vi "Inspection.vi"(8 "Error In":errorcluster, 11 "Data In":T2={"Console log"="", "GUI_Events"={"To_GUI-Producer"=refnum, "To_GUI-Error_message"=refnum, "To_GUI-msg_list"=refnum, "To_GUI-Session"=refnum, "To_GUI-Pre-Session"=refnum, "To_GUI-Consumer"=refnum}, "Function_Queue"={"Queue_MIDI_Handler"=refnum, "Queue_Session"=refnum, "Queue_Producer"=refnum, "Queue_Consumer"=refnum}, "Timout-Time[ms]"=0, "MIDI-Messages"=[], "Com Session State"=enum."Active Session", "Result Data"={"Diff"=[], "Tx Byte"=[], "Rx Byte"=[], "Send Log"=[], "Parsed Data"={"Tx MIDI Tag"=[], "Tx MIDI Parsed Data"=[], "Tx Error"=[], "Tx Running States"=[], "Rx MIDI Tag"=[], "Rx MIDI Parsed Data"=[], "Rx Error"=[], "Rx Running States"=[], "Diff"=[]}}, "Get #"=[], "CPU(ms)"=0}) -> (0 "Error Out":errorcluster, 3 "Consumer Data":T11={"Queue_Consumer"=refnum, "Selected Consumer"=enum."Random", "Session Data"={"Tx-Data"=[], "Rx-Data"=[], "MIDI-Message log"=[{"Message Name"="", "Meta value"=0, "Datastring"="", "Datatype"=enum."No Data"}]}, "Timout-Time[ms]"=0, "To_GUI-Consumer"=refnum, "CPU(ms)"=0, "Console log"="", "MIDI Parse Data"={"MIDI-Bytes In"=[145, 60, 100], "MIDI Tag"=[], "MIDI Parsed Data"=[], "Iteration"=0, "Error?"=[], "Running States"=[], "Running Statusbyte"=0, "Running StatusString"="", "Third Byte Flag"=FALSE, "Current Byte"=0, "Sysex"="", "Expect Databyte"=FALSE}, "Session Inspection Data"={"Diff"=[], "Tx Byte"=[], "Rx Byte"=[], "Send Log"=[], "Parsed Data"={"Tx MIDI Tag"=[], "Tx MIDI Parsed Data"=[], "Tx Error"=[], "Tx Running States"=[], "Rx MIDI Tag"=[], "Rx MIDI Parsed Data"=[], "Rx Error"=[], "Rx Running States"=[], "Diff"=[]}}} {"MIDI Parse Data"."Current Byte" format="%.0x"; "MIDI Parse Data"."Running Statusbyte" format="%.0x"; "MIDI Parse Data"."MIDI-Bytes In" format="%.0x"})   [LabVIEW 2019]
doc: "Description of VI"
uses:
  Common/Controls/Application_Data.ctl
  Common/Controls/App_Events.ctl
  Common/Controls/App_Queues.ctl
  Common/Controls/Application_Message.ctl
  Common/Controls/Application_State.ctl
  MIDI/Controls/MIDI-Message_Array.ctl
  MIDI/Controls/MIDI-Message_Cluster.ctl
  MIDI/Controls/Meta_Commands.ctl
  Producer/Controls/Session_State.ctl
  Controls/Consumer_Result.ctl
  Controls/Parsed_Data.ctl
  Controls/Consumer_Data.ctl
  Controls/Consumer_States.ctl
  Controls/Transfer_Data.ctl
  Controls/Parser-data.ctl
  <vilib>/Utility/error.llb/DialogType.ctl
panel:
  out "Control Tab":T1(tab)
  out "Console Out":string
  out "Error Message":string
  out "VI-filename":string
  out "VI Path":path
  out "Code Size":u32
  out "Revision Number":u32
  in  "Tool Bar:Visible":bool
  in  "Tabs Visible?":bool
  out "VI-Name":string
  # "Add log!"
  # "Settings"
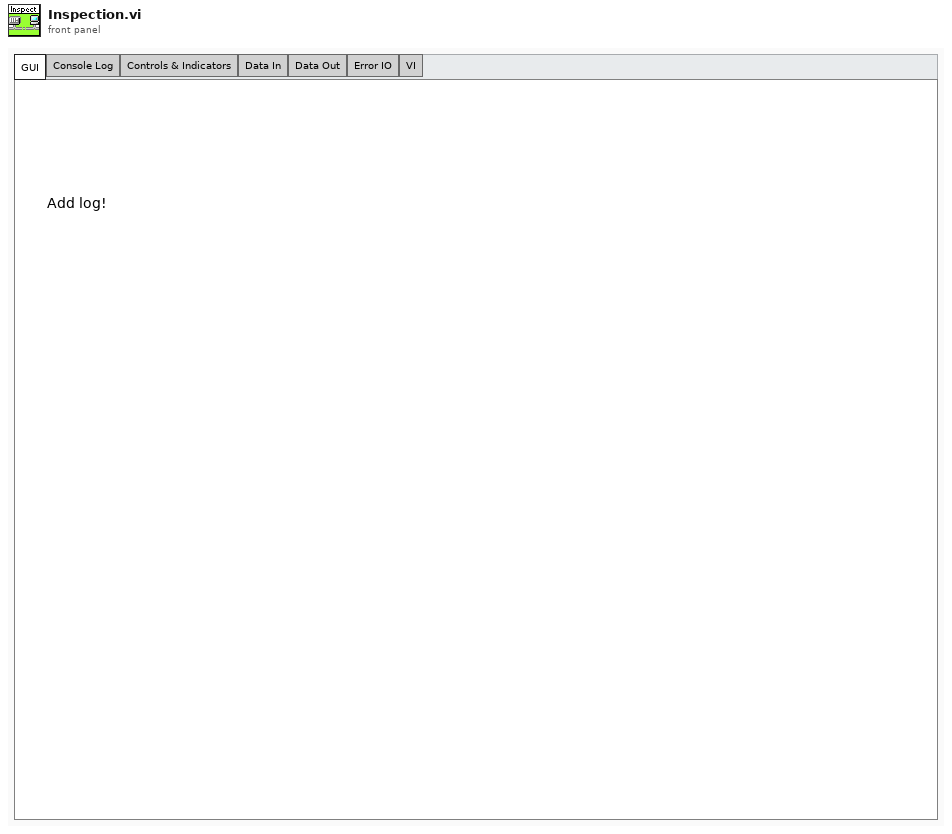
[diagram p1: front panel]
types:
  T1 = enum32{"GUI", "Console Log", "Controls & Indicators", "Data In", "Data Out", "Error IO", "VI"}
  T2 = typedef "Application_Data.ctl" = cluster{"Console log":string, "GUI_Events":T3, "Function_Queue":T4, "Timout-Time[ms]":i32, "MIDI-Messages":T5, "Com Session State":T8, "Result Data":T9, "Get #":bool[], "CPU(ms)":u32}
  T3 = typedef "App_Events.ctl" = cluster{"To_GUI-Producer":refnum<user-event>, "To_GUI-Error_message":refnum<user-event>, "To_GUI-msg_list":refnum<user-event>, "To_GUI-Session":refnum<user-event>, "To_GUI-Pre-Session":refnum<user-event>, "To_GUI-Consumer":refnum<user-event>}
  T4 = typedef "App_Queues.ctl" = cluster{"Queue_MIDI_Handler":refnum<queue>, "Queue_Session":refnum<queue>, "Queue_Producer":refnum<queue>, "Queue_Consumer":refnum<queue>}
  T5 = typedef "MIDI-Message_Array.ctl" = T6[]
  T6 = typedef "MIDI-Message_Cluster.ctl" = cluster{"Message Name":string, "Meta value":i32, "Datastring":string, "Datatype":T7}
  T7 = typedef "Meta_Commands.ctl" = enum16{"No Data", "Pause", "Loop", "Wait for Rx", "Delay", "Break", "MIDI"}
  T8 = typedef "Session_State.ctl" = enum16{"Wait to begin", "Active Session", "Pause", "Wait for Response", "Stop", "Restart", "Inspect", "Exit"}
  T9 = typedef "Consumer_Result.ctl" = cluster{"Diff":bool[], "Tx Byte":string[], "Rx Byte":string[], "Send Log":string[], "Parsed Data":T10}
  T10 = typedef "Parsed_Data.ctl" = cluster{"Tx MIDI Tag":string[], "Tx MIDI Parsed Data":string[], "Tx Error":bool[], "Tx Running States":string[], "Rx MIDI Tag":string[], "Rx MIDI Parsed Data":string[], "Rx Error":bool[], "Rx Running States":string[], "Diff":bool[]}
  T11 = typedef "Consumer_Data.ctl" = cluster{"Queue_Consumer":refnum<queue>, "Selected Consumer":T12, "Session Data":T13, "Timout-Time[ms]":i32, "To_GUI-Consumer":refnum<user-event>, "CPU(ms)":u32, "Console log":string, "MIDI Parse Data":T14, "Session Inspection Data":T9}
  T12 = typedef "Consumer_States.ctl" = enum16{"Random", "ECG", "Strech-Patch"}
  T13 = typedef "Transfer_Data.ctl" = cluster{"Tx-Data":i8[], "Rx-Data":i8[], "MIDI-Message log":T5}
  T14 = typedef "Parser-data.ctl" = cluster{"MIDI-Bytes In":u8[], "MIDI Tag":string[], "MIDI Parsed Data":string[], "Iteration":i32, "Error?":bool[], "Running States":string[], "Running Statusbyte":u8, "Running StatusString":string, "Third Byte Flag":bool, "Current Byte":u8, "Sysex":string, "Expect Databyte":bool}
  T15 = typedef "DialogType.ctl" = u16
  T16 = enum16{"open", "replace", "create", "open or create", "replace or create", "replace or create with confirmation"}
  T17 = typedef "Application_State.ctl" = enum16{"Idle", "Initiate", "MH Load Messages", "Prepare for Tx", "Settings", "Com Session", "Receive", "Data", "Uninitialize", "Quit Message", "Export Send"}
  T18 = typedef "Application_Message.ctl" = cluster{"Application State":T17, "Payload":variant}
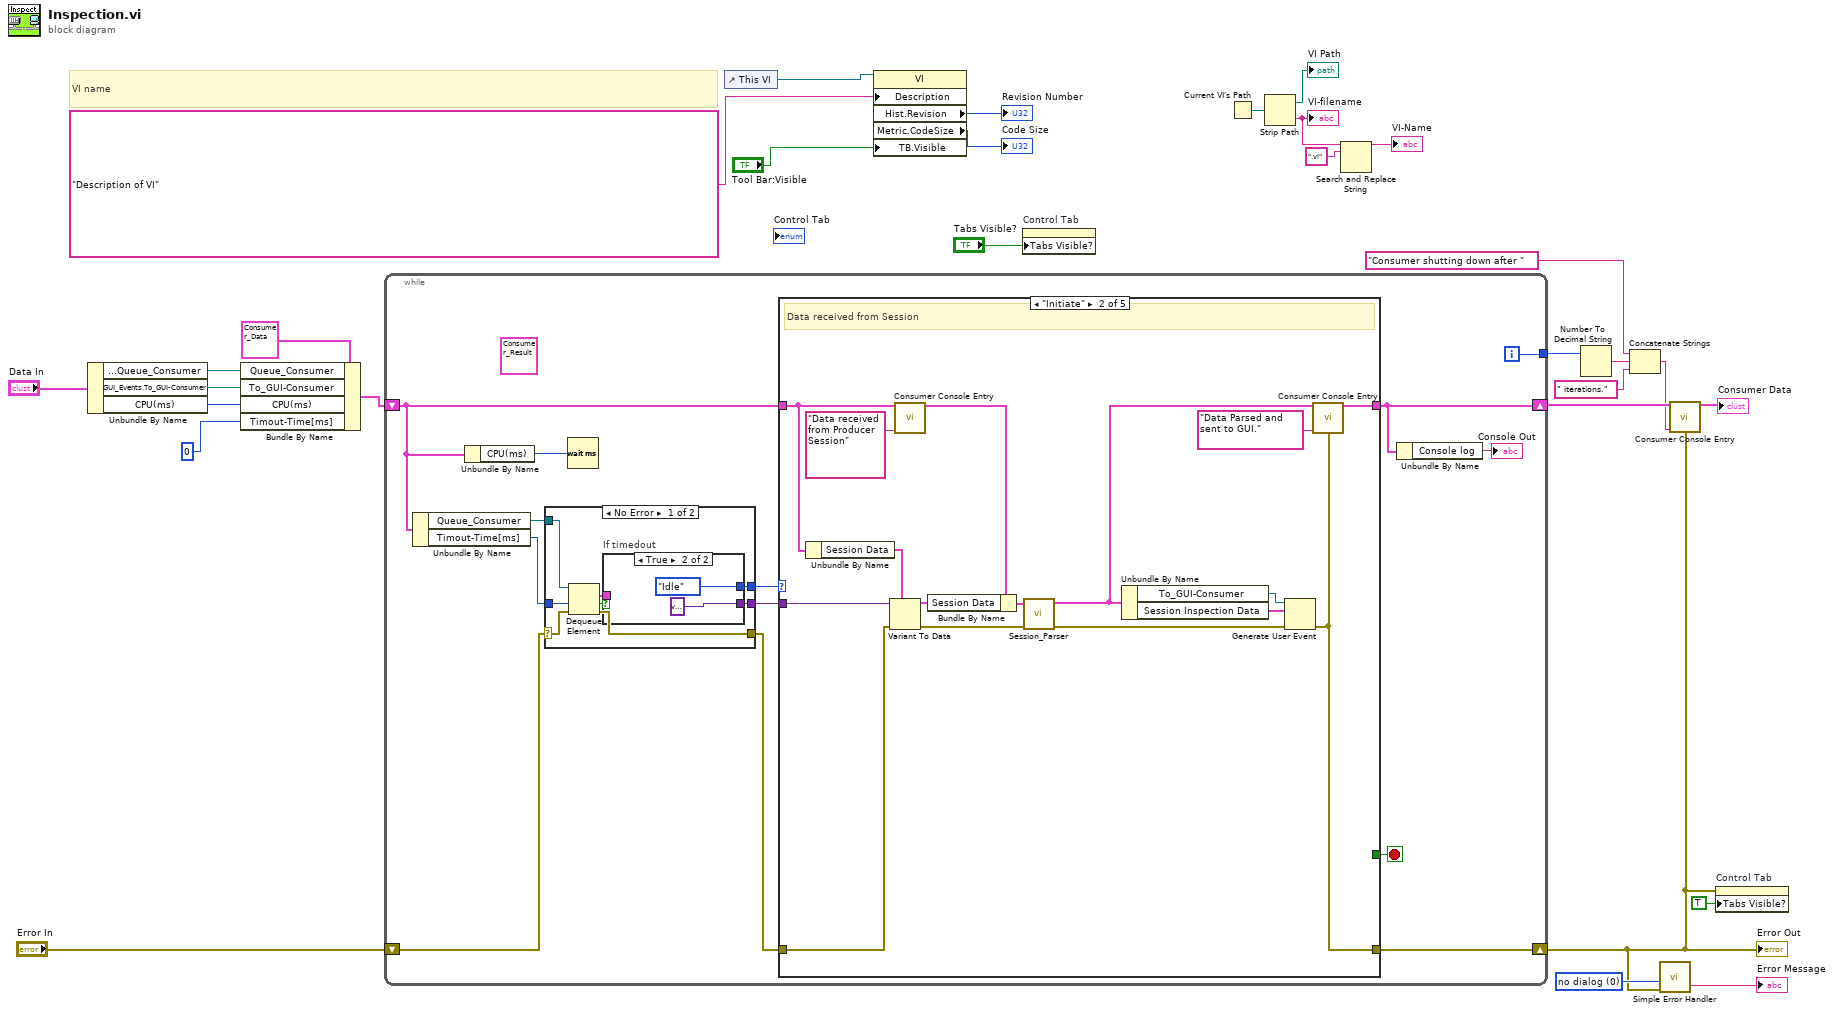
[diagram p0: block diagram]
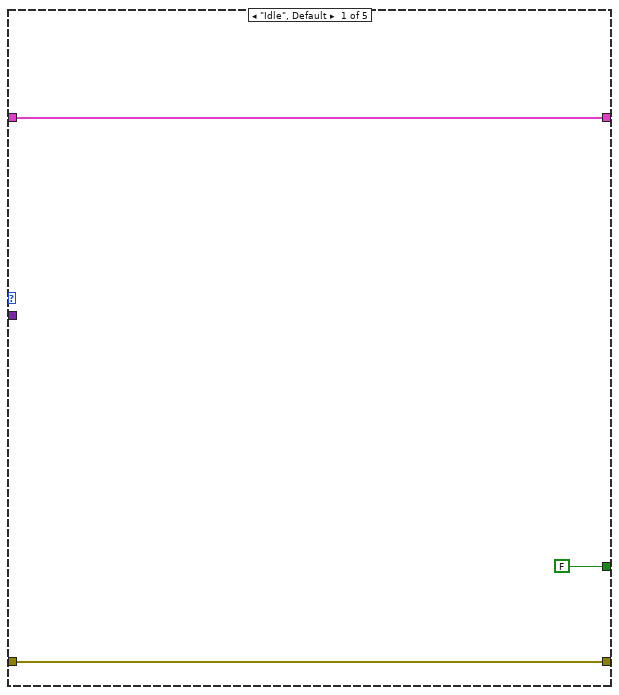
[diagram p2: hidden frame]
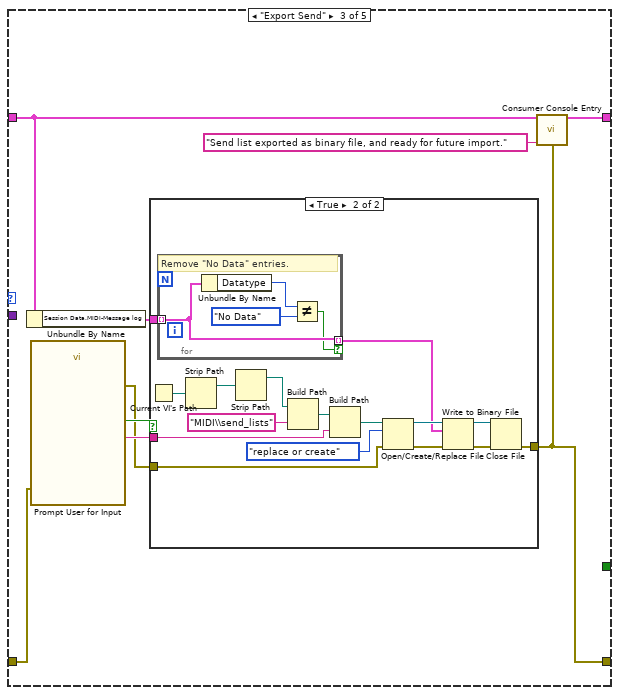
[diagram p3: hidden frame]
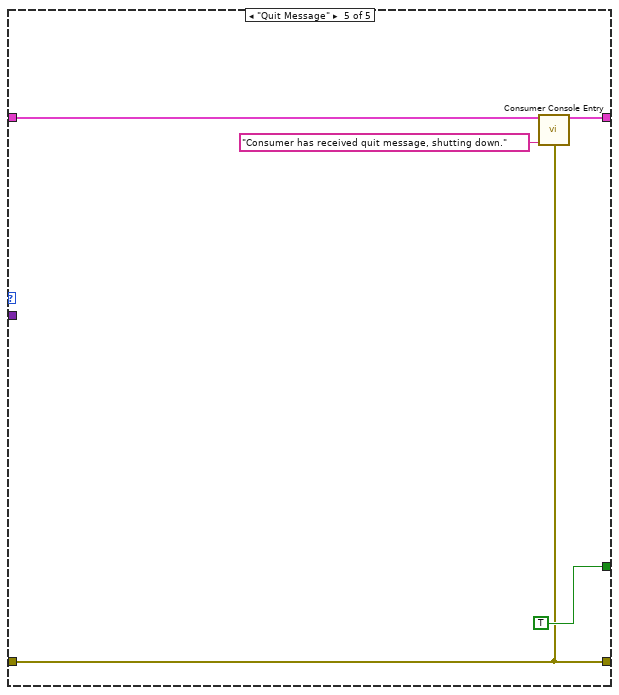
[diagram p6: hidden frame]
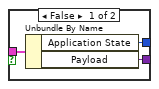
[diagram p7: hidden frame]
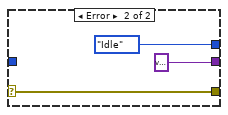
[diagram p8: hidden frame]
diagram:
  w21 = T15 0 items=["no dialog", "OK message", "continue or stop message", "OK message + warnings", "continue/stop + warnings"] ("type of dialog (OK msg:1)")
  # "VI name"
  n1 = Unbundle By Name("Data In") -> ("Function_Queue.Queue_Consumer"=w14:refnum<queue>, "GUI_Events.To_GUI-Consumer"=w11:refnum<user-event>, "CPU(ms)"=w9:u32)
  n2 = Bundle By Name(cluster=T11 {"Queue_Consumer"=refnum, "Selected Consumer"=enum."Random", "Session Data"={"Tx-Data"=[], "Rx-Data"=[], "MIDI-Message log"=[{"Message Name"="", "Meta value"=0, "Datastring"="", "Datatype"=enum."No Data"}]}, "Timout-Time[ms]"=0, "To_GUI-Consumer"=refnum, "CPU(ms)"=0, "Console log"="", "MIDI Parse Data"={"MIDI-Bytes In"=[145, 60, 100], "MIDI Tag"=[], "MIDI Parsed Data"=[], "Iteration"=0, "Error?"=[], "Running States"=[], "Running Statusbyte"=0, "Running StatusString"="", "Third Byte Flag"=FALSE, "Current Byte"=0, "Sysex"="", "Expect Databyte"=FALSE}, "Session Inspection Data"={"Diff"=[], "Tx Byte"=[], "Rx Byte"=[], "Send Log"=[], "Parsed Data"={"Tx MIDI Tag"=[], "Tx MIDI Parsed Data"=[], "Tx Error"=[], "Tx Running States"=[], "Rx MIDI Tag"=[], "Rx MIDI Parsed Data"=[], "Rx Error"=[], "Rx Running States"=[], "Diff"=[]}}} ("Consumer Data"), "Queue_Consumer"=w14, "To_GUI-Consumer"=w11, "CPU(ms)"=w9, "Timout-Time[ms]"=0) -> (w13:T11)
  n3 = while {
    shift-right: [w33] -> w7
    shift-left: w13 -> [w35]
    shift-right: [w38] -> w1
    shift-left: "Error In" -> [w40]
    tunnel: [w31] -> w4
    i -> [w31]
    stop <- w36 stop-if-true
    (unwired) T9 {"Diff"=[], "Tx Byte"=[], "Rx Byte"=[], "Send Log"=[], "Parsed Data"={"Tx MIDI Tag"=[], "Tx MIDI Parsed Data"=[], "Tx Error"=[], "Tx Running States"=[], "Rx MIDI Tag"=[], "Rx MIDI Parsed Data"=[], "Rx Error"=[], "Rx Running States"=[], "Diff"=[]}}
    n4 = Unbundle By Name(w35) -> ("Queue_Consumer"=w43:refnum<queue>, "Timout-Time[ms]"=w42:i32)
    n5 = Unbundle By Name(w35) -> ("CPU(ms)"=w34:u32)
    n6 = case shown="No Error" w40 {
      selector: w40 -> [w104 w115]
      tunnel: [w103 w115] -> w39
      tunnel: [w106 Application_State."Idle" ("Data_Type")] -> w41
      tunnel: [w105 variant ("Payload")] -> w37
      tunnel: w43 -> [w102 _]
      tunnel: w42 -> [w101 _]
      frame No Error {
        n7 = Dequeue Element(queue=w102, timeout in ms (-1)=w101, error in (no error)=w104) -> (element=w107:T18, timed out?=w100:bool, error out=w103:errorcluster)  [unwired: 1 out]
        n8 = case "If timedout" shown="True" w100 {
          tunnel: w107 -> [w110 _]
          tunnel: [w109 Application_State."Idle" ("Data_Type")] -> w106
          tunnel: [w108 variant ("Payload")] -> w105
          frame False {
            n9 = Unbundle By Name(w110) -> ("Application State"=w109:T17, "Payload"=w108:variant)
          }
          frame True {
          }
        }
      }
      frame Error {
      }
    }
    n10 = Wait (ms)(milliseconds to wait=w34) -> ()  [unwired: 1 out]
    n11 = case shown="\"Initiate\"" w41 {
      tunnel: w35 -> [w46 w50 w65 w94 w97]
      tunnel: w39 -> [w45 w60 w70 w93 w96]
      tunnel: [w45 w47 w64 w93 w96] -> w38
      tunnel: w37 -> [_ w62 _ _ _]
      tunnel: [w46 w53 w66 w94 w98] -> w33
      tunnel: [FALSE _ _ _ TRUE] -> w36
      frame "Idle", Default {
      }
      frame "Initiate" {
        # "Data received from Session"
        n12 = Unbundle By Name(w50) -> ("Session Data"=w61:T13)
        n13 = Variant To Data(error in=w60, type=w61, Variant=w62) -> (data=w59:T13, error out=w57:errorcluster)
        n14 = call "Consumer Console Entry.vi"("Consumer Data In"=w50, "Console Entry"="Data received from Producer Session") -> ("Consumer Data Out"=w49:T11)  [unwired: 13 in]
        n15 = Bundle By Name(cluster=w49, "Session Data"=w59) -> (w58:T11)
        n16 = call "Session_Parser.vi"("Error In"=w57, "Consumer Data In"=w58) -> ("Error Out"=w54:errorcluster, "Consumer Data Out"=w52:T11)  [unwired: 8 in]
        n17 = Unbundle By Name(w52) -> ("To_GUI-Consumer"=w56:refnum<user-event>, "Session Inspection Data"=w55:T9)
        n18 = Generate User Event(user event=w56, event data cluster=w55, error in=w54) -> (error out=w47:errorcluster)  [unwired: 1 in, 1 out]
        n19 = call "Consumer Console Entry.vi"("Consumer Data In"=w52, "Console Entry"="Data Parsed and sent to GUI.", "Error In"=w47) -> ("Consumer Data Out"=w53:T11)  [unwired: 12 in]
      }
      frame "Export Send" {
        n20 = Unbundle By Name(w65) -> ("Session Data.MIDI-Message log"=w67:T5)
        n21 = call "Prompt User for Input"("error in (no error)"=w70) -> ("Filename"=w71:string, "Save"=w69:bool, "error out"=w68:errorcluster)  [unwired: 16 in]
        n22 = case shown="True" w69 {
          tunnel: w71 -> [_ w83]
          tunnel: w68 -> [w72 w80]
          tunnel: [w72 w75] -> w64
          tunnel: w67 -> [_ w74]
          frame False {
          }
          frame True {
            n23 = Current VI's Path() -> (path=w87:path)
            n24 = for {
              tunnel: w74 -> [w92] mode=indexing
              tunnel: [w92] -> w73 mode=indexing if=w89
              # "Remove \"No Data\" entries."
              n25 = Unbundle By Name(w92) -> ("Datatype"=w91:T7)
              n26 = Not Equal?(x=w91, y=Meta_Commands."No Data") -> (x != y?=w89:bool)
            }
            n27 = Strip Path(path=w87) -> (stripped path=w88:path)  [unwired: 1 out]
            n28 = Strip Path(path=w88) -> (stripped path=w86:path)  [unwired: 1 out]
            n29 = Build Path(base path=w86, name or relative path="MIDI\\send_lists") -> (appended path=w84:path)
            n30 = Build Path(base path=w84, name or relative path=w83) -> (appended path=w82:path)
            n31 = Open/Create/Replace File(file path (use dialog)=w82, error in=w80, operation (0:open)=T16."replace or create") -> (refnum out=w78:refnum<file>, error out=w79:errorcluster)  [unwired: 3 in, 1 out]
            n32 = Write to Binary File(file (use dialog)=w78, data=w73, error in=w79) -> (refnum out=w76:refnum<file>, error out=w77:errorcluster)  [unwired: 3 in, 1 out]
            n33 = Close File(refnum=w76, error in=w77) -> (error out=w75:errorcluster)  [unwired: 1 out]
          }
        }
        n34 = call "Consumer Console Entry.vi"("Consumer Data In"=w65, "Console Entry"="Send list exported as binary file, and ready for future import.", "Error In"=w64) -> ("Consumer Data Out"=w66:T11)  [unwired: 12 in]
      }
      frame "Data" {
      }
      frame "Quit Message" {
        n35 = call "Consumer Console Entry.vi"("Consumer Data In"=w97, "Console Entry"="Consumer has received quit message, shutting down.", "Error In"=w96) -> ("Consumer Data Out"=w98:T11)  [unwired: 12 in]
      }
    }
    n36 = Unbundle By Name(w33) -> ("Console log"=→"Console Out":string)
  }
  "Error Out" <- w1
  n37 = control-ref of="This VI"() -> (w27:refnum<vi>)
  n38 = property class="VI"(reference=w27, "Description"="Description of VI", "TB.Visible"="Tool Bar:Visible") -> ("Hist.Revision"=→"Revision Number":u32, "Metric.CodeSize"=→"Code Size":u32)  [unwired: 1 in, 2 out]
  n39 = property on="Control Tab" class="TabCtl (strict)"("Tabs Visible?"="Tabs Visible?") -> ()  [unwired: 2 in, 2 out]
  n40 = Current VI's Path() -> (path=w30:path)
  n41 = Strip Path(path=w30) -> (stripped path=→"VI Path":path, name=w24:string)
  "VI-filename" <- w24
  n42 = Search and Replace String(input string=w24, search string=".vi") -> (result string=→"VI-Name":string)  [unwired: 6 in, 3 out]
  n43 = Number To Decimal String(number=w4) -> (decimal integer string=w6:string)  [unwired: 1 in]
  n44 = Concatenate Strings("Consumer shutting down after " ("string"), w6, " iterations." ("string")) -> (w2:string)
  n45 = call <vilib>:"Simple Error Handler.vi"("type of dialog (OK msg:1)"=w21, "error in (no error)"=w1) -> ("message"=→"Error Message":string)  [unwired: 3 in, 4 out]
  n46 = call "Consumer Console Entry.vi"("Consumer Data In"=w7, "Console Entry"=w2, "Error In"=w1) -> ("Consumer Data Out"=→"Consumer Data":T11)  [unwired: 12 in]
  n47 = property on="Control Tab" class="TabCtl (strict)"(error in=w1, "Tabs Visible?"=TRUE) -> ()  [unwired: 1 in, 2 out]
